vi "arb_config.vi"(8 "error in (no error)":errorcluster, 9 "name":string="ADAM1", 10 "output":T1={"rate (Sa / s)"=20000000.0, "amp (V)"=0.1, "offset (V)"=0.0}, 11 "chan":i32(ring)=1 items=["1"=1, "2"=2]) -> (0 "error out":errorcluster, 2 "cmd":string="SOUR1:FUNC ARB;\nSOUR1:FUNC:ARB ADAM1;\nSOUR1:FUNC:ARB:FILT OFF;\nSOUR1:FUNC:ARB:SRAT 2E+7;\nSOUR1:VOLT 0.1;\nSOUR1:VOLT:OFFS 0;")   [LabVIEW 2017, in "wf.lvlib"]
uses:
  wf.lvlib
  wf_output.ctl
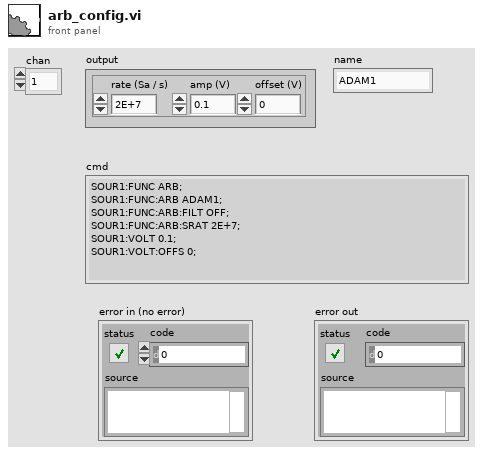
[diagram p1: front panel]
types:
  T1 = typedef "wf.lvlib/wf_output.ctl" = cluster{"rate (Sa / s)":dbl, "amp (V)":dbl, "offset (V)":dbl}
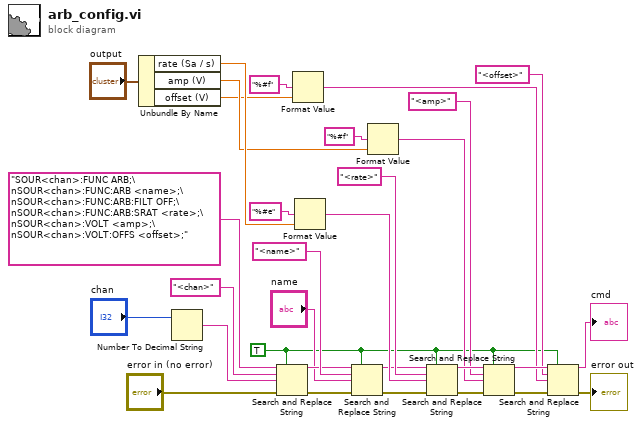
[diagram p0: block diagram]
diagram:
  w1 = TRUE ("replace all? (F)")
  n1 = Unbundle By Name("output") -> ("rate (Sa / s)"=w16:dbl, "amp (V)"=w15:dbl, "offset (V)"=w12:dbl)
  n2 = Number To Decimal String(number="chan") -> (decimal integer string=w31:string)  [unwired: 1 in]
  n3 = Search and Replace String(replace all?=w1, input string="SOUR<chan>:FUNC ARB;\nSOUR<chan>:FUNC:ARB <name>;\nSOUR<chan>:FUNC:ARB:FILT OFF;\nSOUR<chan>:FUNC:ARB:SRAT <rate>;\nSOUR<chan>:VOLT <amp>;\nSOUR<chan>:VOLT:OFFS <offset>;", search string="<chan>", replace string=w31, error in="error in (no error)") -> (result string=w22:string, error out=w24:errorcluster)  [unwired: 3 in, 2 out]
  n4 = Format Value(format string="%#f", value (0)=w12) -> (output string=w10:string)  [unwired: 1 in]
  n5 = Format Value(format string="%#e", value (0)=w16) -> (output string=w29:string)  [unwired: 1 in]
  n6 = Search and Replace String(replace all?=w1, input string=w22, search string="<name>", replace string="name", error in=w24) -> (result string=w25:string, error out=w27:errorcluster)  [unwired: 3 in, 2 out]
  n7 = Format Value(format string="%#f", value (0)=w15) -> (output string=w17:string)  [unwired: 1 in]
  n8 = Search and Replace String(replace all?=w1, input string=w25, search string="<rate>", replace string=w29, error in=w27) -> (result string=w20:string, error out=w6:errorcluster)  [unwired: 3 in, 2 out]
  n9 = Search and Replace String(replace all?=w1, input string=w20, search string="<amp>", replace string=w17, error in=w6) -> (result string=w14:string, error out=w5:errorcluster)  [unwired: 3 in, 2 out]
  n10 = Search and Replace String(replace all?=w1, input string=w14, search string="<offset>", replace string=w10, error in=w5) -> (result string=→"cmd":string, error out=→"error out":errorcluster)  [unwired: 3 in, 2 out]
